vi "Start Round.vi"(10 "Round":u32, 11 "Team in":refnum<class "Team.lvclass">) -> (3 "Team out":refnum<class "Team.lvclass">)   [LabVIEW 2020, in "SquareBattle.lvlib" / "Team.lvclass"]
uses:
  Team.lvclass
  Team.lvclass/Team.ctl
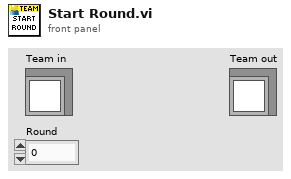
[diagram p1: front panel]
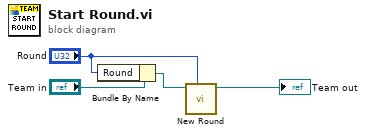
[diagram p0: block diagram]
diagram:
  n1 = Bundle By Name(cluster="Team in", "Round"="Round") -> (w3:refnum<class "Team.lvclass">)
  n2 = call-dynamic "New Round.vi"("Round"="Round", "Team in"=w3) -> ("Team out"=→"Team out":refnum<class "Team.lvclass">)  [unwired: 9 in]
